vi "PDLM_DecodeSystemStatus.vi"(8 "error in (no error)":errorcluster, 10 "state":u32) -> (0 "error out":errorcluster, 2 "Buffer":string, 3 "return type":i32)   [LabVIEW 2019]
uses:
  <userlib>/TaikoLaser/PDLM_DllPath_global.vi
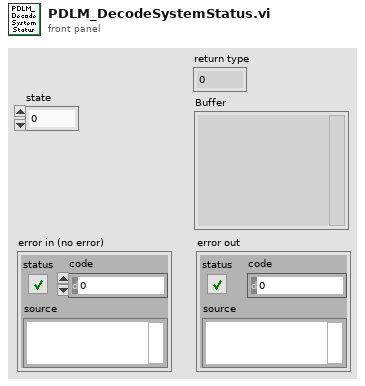
[diagram p1: front panel]
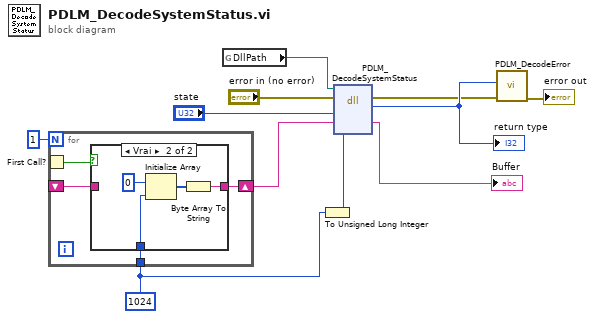
[diagram p0: block diagram]
diagram:
  w1 = 1024 ("dimension size")
  n1 = for {
    N: 1 -> [_]
    shift-right: [w14] -> w2
    shift-left: _ -> [w13]
    tunnel: w1 -> [w12]
    n2 = First Call?() -> (First Call?: T/F=w15:bool)
    n3 = case shown="Vrai" w15 {
      tunnel: [w16 w18] -> w14
      tunnel: w13 -> [w16 _]
      tunnel: w12 -> [_ w17]
      frame False {
      }
      frame True {
        n4 = Initialize Array(u8 0, w17) -> (w19:u8[])
        n5 = Byte Array To String(unsigned byte array=w19) -> (string=w18:string)
      }
    }
  }
  n6 = global read "PDLM_DllPath_global.vi" "DllPath"() -> (w7:path)
  n7 = To Unsigned Long Integer(number=w1) -> (unsigned 32bit integer=w5:u32)
  n8 = dll-call lib="M:/_dev/progs/LabVIEW/_lib/PQ/Taiko/pdlm_lib.dll" fn="PDLM_DecodeSystemStatus"(path in=w7, error in="error in (no error)", "state"="state", "Buffer"=w2, "BuffLen"=w5) -> (error out=w9:errorcluster, "return type"=w10:i32, "Buffer"=→"Buffer":string)  [unwired: 3 in, 1 out]
  "return type" <- w10
  n9 = call <userlib>:"PDLM_DecodeError.vi"("error in (no error)"=w9, "code"=w10) -> ("error out"=→"error out":errorcluster)  [unwired: 7 in, 2 out]
